vi "Next Step.vi"(8 "error in (no error)":errorcluster, 11 "Microwave Freq Scan in":refnum<class "Microwave Freq Scan.lvclass">) -> (0 "error out":errorcluster, 1 "Current Step":u32, 2 "Current Position":dbl, 3 "Microwave Freq Scan out":refnum<class "Microwave Freq Scan.lvclass">)   [LabVIEW 2017, in "Microwave Freq Scan.lvclass"]
doc: "(Dynamic) Move to the next preconfigured step of this Scanner, and return the current position (actual, not intended) of this Scanner. Increment the step counter by one."
uses:
  Microwave Freq Scan.lvclass
  Scanner/Scanner.lvclass
  Instruments/Utility Classes/Scannable/Scannable.lvclass
  Instruments/Microwave/Agilent PSG MXG Series/Agilent PSG MXG Series.lvlib
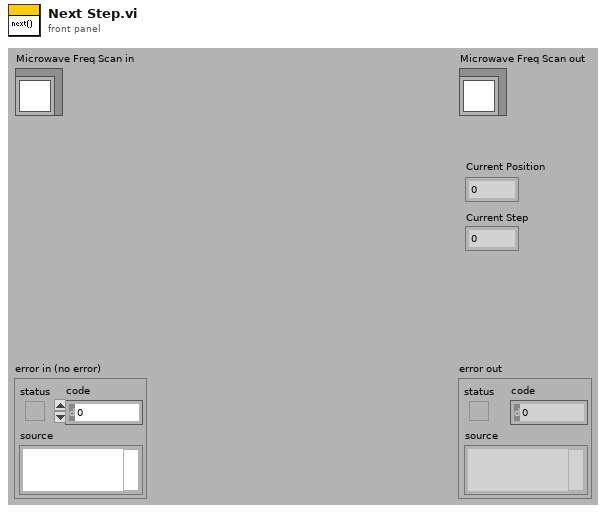
[diagram p1: front panel]
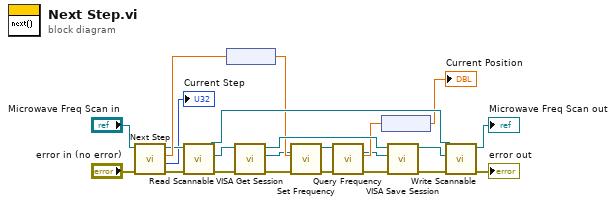
[diagram p0: block diagram]
diagram:
  n1 = call-parent "Next Step.vi"("error in (no error)"="error in (no error)", "Scanner in"="Microwave Freq Scan in") -> ("error out"=w14:errorcluster, "Current Step"=→"Current Step":u32, "Current Position"=w10:dbl, "Scanner out"=w8:refnum<class "Microwave Freq Scan.lvclass">)  [unwired: 6 out]
  n2 = call-dynamic "Read Scannable.vi"("error in (no error)"=w14, "Scanner.lvclass in"=w8) -> ("error out"=w13:errorcluster, "Scannable.lvclass"=w9:refnum<class "Scannable.lvclass">, "Scanner.lvclass out"=w21:refnum<class "Microwave Freq Scan.lvclass">)  [unwired: 7 out]
  n3 = node(w10) -> (w11:dbl[unit])
  n4 = call-dynamic "VISA Get Session.vi"("error in (no error)"=w13, "Instrument.lvclass in"=w9) -> ("error out"=w12:errorcluster, "VISA Resource Name"=w4:refnum<visa-resource-name>, "Instrument.lvclass out"=w20:refnum<class "Scannable.lvclass">)  [unwired: 7 out]
  n5 = call "Set Frequency.vi"("error in (no error)"=w12, "Frequency"=w11, "VISA resource name"=w4) -> ("error out"=w16:errorcluster, "VISA resource name out"=w15:refnum<visa-resource-name>)  [unwired: 7 out]
  n6 = call "Query Frequency.vi"("error in (no error)"=w16, "VISA resource name"=w15) -> ("error out"=w18:errorcluster, "Frequency"=w19:dbl[unit], "VISA resource name out"=w17:refnum<visa-resource-name>)  [unwired: 7 out]
  n7 = node(w19) -> (→"Current Position":dbl)
  n8 = call-dynamic "VISA Save Session.vi"("error in (no error)"=w18, "VISA Resource Name"=w17, "Instrument.lvclass in"=w20) -> ("error out"=w23:errorcluster, "Instrument.lvclass out"=w22:refnum<class "Scannable.lvclass">)  [unwired: 7 out]
  n9 = call-dynamic "Write Scannable.vi"("error in (no error)"=w23, "Scannable.lvclass"=w22, "Scanner.lvclass in"=w21) -> ("error out"=→"error out":errorcluster, "Scanner.lvclass out"=→"Microwave Freq Scan out":refnum<class "Microwave Freq Scan.lvclass">)  [unwired: 7 out]
